vi "test-ltv-differential-drive-controller-dynamics.vi"(9 "U":T1, 10 "X":T1, 11 "Info":variant) -> (0 "Error":bool, 3 "XDOT":T1)   [LabVIEW 2019]
uses:
  <vilib>/Analysis/Matrix/Datatypes/RealMatrix.ctl
  <vilib>/Analysis/baseanly.llb/Real A x B.vi
  <vilib>/Rock Robotics/WPI/ThirdParty/JAS_Junk/TrajLib/MatrixHelper_CoerceSize.vi
  <vilib>/Rock Robotics/WPI/ThirdParty/JAS_Junk/TrajLib/MatBuilder_Create.vi
  <vilib>/Analysis/Matrix/Numeric/Add/Add - RM,RM.vi
  <vilib>/Rock Robotics/WPI/ThirdParty/JAS_Junk/TrajLib/Trajectory_Library.lvlib
  <vilib>/Analysis/NI_AALBase.lvlib
  <vilib>/Analysis/Matrix/NI_Matrix.lvlib
panel:
  in  "Cluster":cluster{"A":T1, "B":T1}
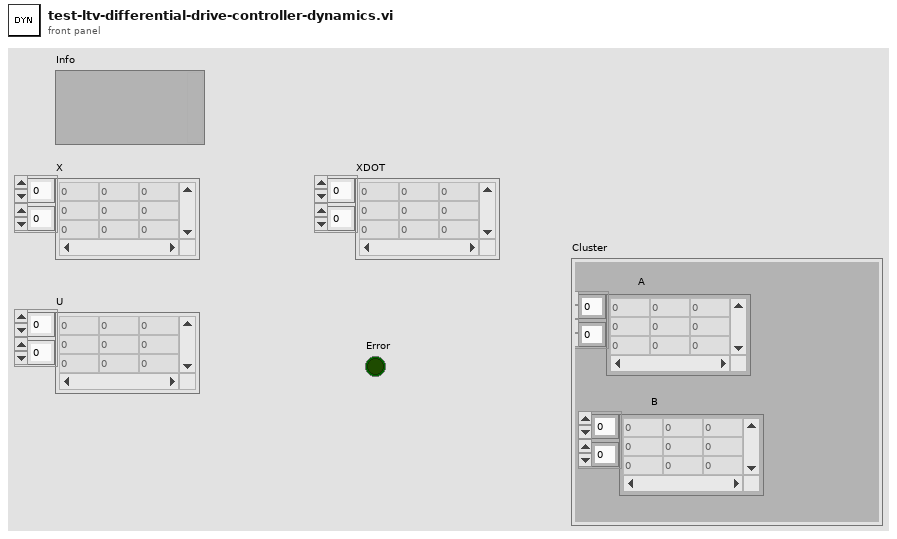
[diagram p1: front panel]
types:
  T1 = typedef "NI_Matrix.lvlib/RealMatrix.ctl" = dbl[][]
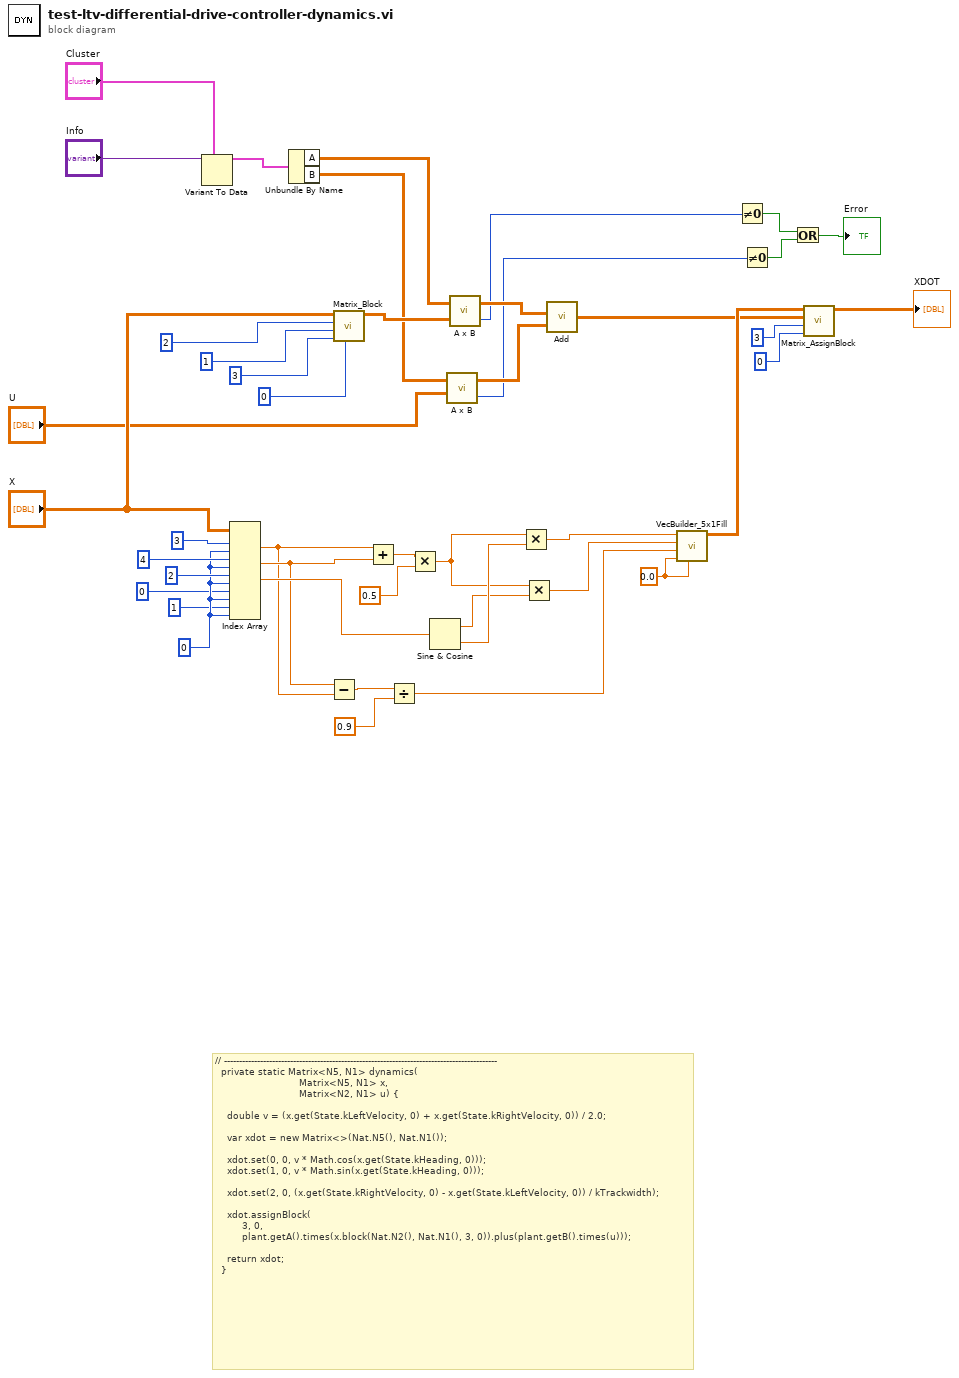
[diagram p0: block diagram]
diagram:
  w8 = 0.0 ("R3")
  w33 = 0 ("index (col)")
  # "// -------------------------------------------------------------------------------------------\n  private static Matrix<N5, N1> dynamics(\n                            Matrix<N5, N1> x, \n                            Matrix<N2, N1> u) {\n\n    double v = (x.get(State.kLeftVelocity, 0) + x.get(State.kRightVelocity, 0)) / 2.0;\n\n    var xdot = new Matrix<>(Nat.N5(), Nat.N1());\n\n    xdot.set(0, 0, v * Math.cos(x.get(State.kHeading, 0)));\n    xdot.set(1, 0, v * Math.sin(x.get(State.kHeading, 0)));\n\n    xdot.set(2, 0, (x.get(State.kRightVelocity, 0) - x.get(State.kLeftVelocity, 0)) / kTrackwidth);\n\n    xdot.assignBlock(\n         3, 0, \n         plant.getA().times(x.block(Nat.N2(), Nat.N1(), 3, 0)).plus(plant.getB().times(u)));\n\n    return xdot;\n  }"
  n1 = Variant To Data(type="Cluster", Variant="Info") -> (data=w25:cluster{"A":T1, "B":T1})  [unwired: 1 in, 1 out]
  n2 = Index Array(array="X", index (row) #1=3 ("index (row)"), index (col) #1=w33, index (row) #2=4 ("index (row)"), index (col) #2=w33, index (row) #3=2 ("index (row)"), index (col) #3=w33, index (row) #4=0 ("index (row)"), index (col) #4=w33, index (row) #5=1 ("index (row)"), index (col) #5=w33) -> (element #1=w1:dbl, element #2=w2:dbl, element #3=w39:dbl)  [unwired: 2 out]
  n3 = Unbundle By Name(w25) -> ("A"=w18:T1, "B"=w17:T1)
  n4 = Subtract(x=w2, y=w1) -> (x-y=w30:dbl)
  n5 = call <vilib>:"Matrix_Block.vi"("StartColumn"=0, "StartRow"=3, "Columns"=1, "Rows"=2, "input matrix"="X") -> ("output matrix"=w19:T1)  [unwired: 6 in]
  n6 = Add(x=w1, y=w2) -> (x+y=w42:dbl)
  n7 = Divide(x=w30, y=0.9) -> (x/y=w28:dbl)
  n8 = Multiply(x=w42, y=0.5) -> (x*y=w36:dbl)
  n9 = Sine & Cosine(0:w39) -> (1:w37:dbl, 2:w38:dbl)
  n10 = call-poly <vilib>:"A x B.vi"("B"="U", "A"=w17) -> ("error"=w9:i32, "A x B"=w14:T1)
  n11 = call-poly <vilib>:"A x B.vi"("B"=w19, "A"=w18) -> ("error"=w10:i32, "A x B"=w15:T1)
  n12 = Multiply(x=w36, y=w38) -> (x*y=w35:dbl)
  n13 = Multiply(x=w36, y=w37) -> (x*y=w34:dbl)
  n14 = call-poly <vilib>:"Add.vi"("Real Matrix B"=w14, "Real Matrix A"=w15) -> ("A + B"=w6:T1)
  n15 = call <vilib>:"VecBuilder_5x1Fill.vi"("R4"=w8, "R3"=w8, "R2"=w28, "R1"=w34, "R0"=w35) -> ("output matrix"=w7:T1)  [unwired: 6 in]
  n16 = Not Equal To 0?(x=w10) -> (x != 0?=w12:bool)
  n17 = Not Equal To 0?(x=w9) -> (x != 0?=w11:bool)
  n18 = Or(x=w12, y=w11) -> (x .or. y?=→"Error":bool)
  n19 = call <vilib>:"Matrix_AssignBlock.vi"("StartColumn"=0, "StartRow"=3, "Other Matrix"=w6, "input matrix"=w7) -> ("output matrix"=→"XDOT":T1)  [unwired: 7 in]
